vi "FullAlign.vi"(0 "Joystick 0":dbl, 1 "Button":bool=TRUE, 5 "Joystick 1":dbl, 7 "Distance":dbl=23.73829999999998, 9 "Angle":dbl=57.28800997198897) -> (4 "Right Motor":dbl, 6 "Left Motor":dbl=-0.0, 15 "In Range?":bool)   [LabVIEW 2016]
panel:
  in  "Range":dbl=25.0 step=5.0 format="%#_13g"
  out "Sees Target?":bool=TRUE
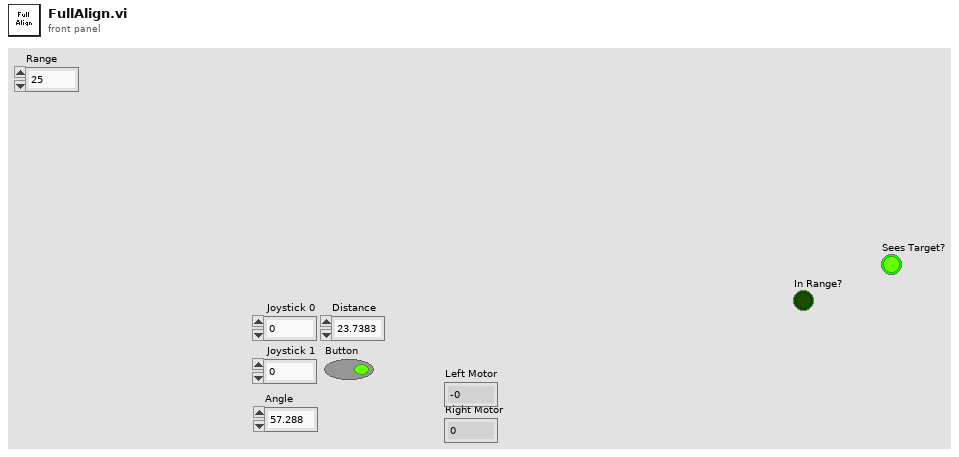
[diagram p1: front panel]
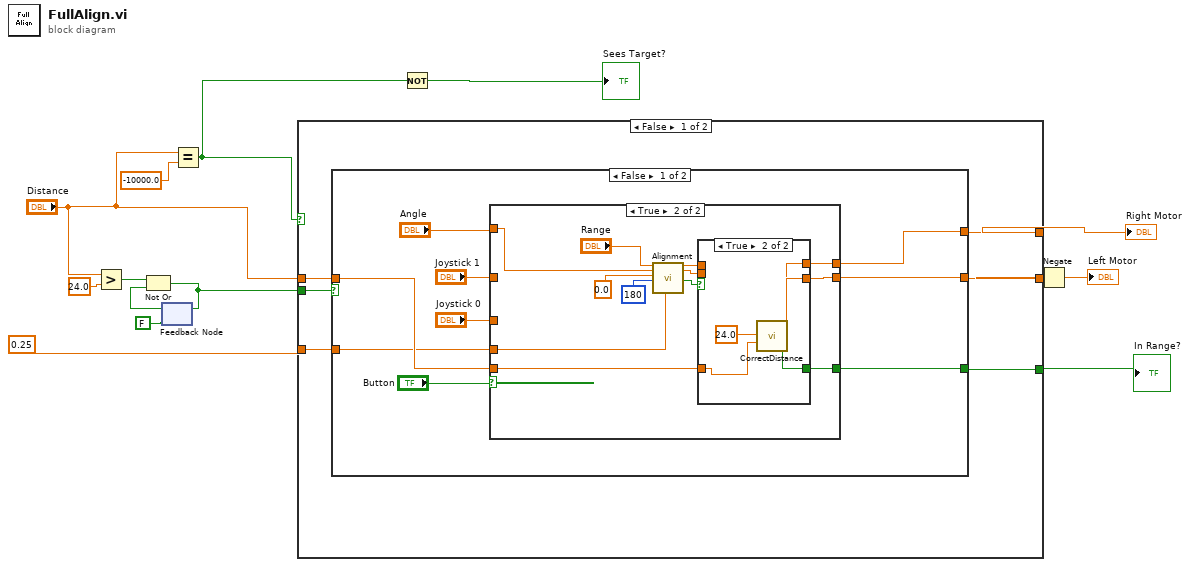
[diagram p0: block diagram]
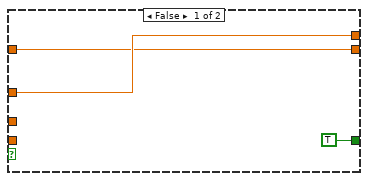
[diagram p2: hidden frame]
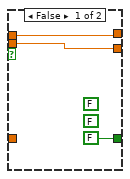
[diagram p3: hidden frame]
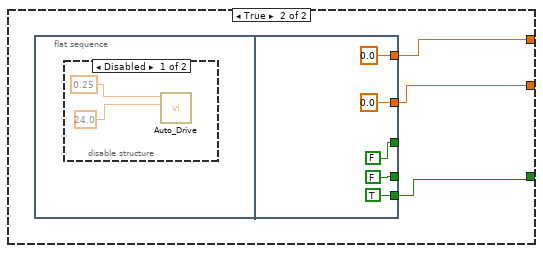
[diagram p4: hidden frame]
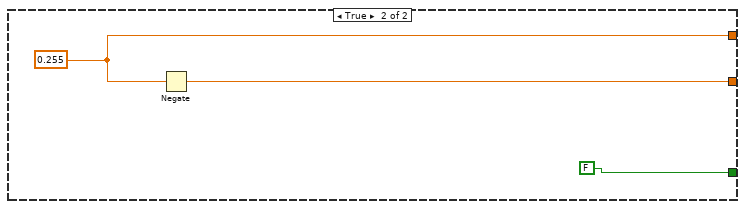
[diagram p6: hidden frame]
diagram:
  n1 = Greater?(x="Distance", y=24.0) -> (0:w11:bool)
  n2 = feedback #1(FALSE) -> (w12:bool)
  n3 = Not Or(1:w12, 2:w11) -> (0:w10:bool)
  n4 = feedback-in #1(w10) -> ()
  n5 = Equal?(x="Distance", y=-10000.0) -> (x = y?=w7:bool)
  n6 = case shown="False" w7 {
    tunnel: w10 -> [w20 _]
    tunnel: [w19 w63] -> w3
    tunnel: [w18 w64] -> w4
    tunnel: [w17 FALSE] -> w9
    tunnel: "Distance" -> [w16 _]
    tunnel: 0.25 -> [w15 _]
    frame False {
      n7 = case shown="False" w20 {
        tunnel: w16 -> [w25 _]
        tunnel: [w24 w54] -> w19
        tunnel: [w23 w53] -> w18
        tunnel: [w22 w55] -> w17
        tunnel: w15 -> [w21 _]
        frame False {
          n8 = case shown="True" "Button" {
            tunnel: "Joystick 1" -> [w31 _]
            tunnel: "Joystick 0" -> [w32 _]
            tunnel: [w31 w44] -> w23
            tunnel: [w32 w43] -> w24
            tunnel: "Angle" -> [_ w37]
            tunnel: [TRUE w42] -> w22
            tunnel: w25 -> [_ w41]
            tunnel: w21 -> [_ w36]
            frame False {
            }
            frame True {
              n9 = call "Alignment.vi"("Range"="Range", "Camera Feedback"=w37, "Target"=0.0, "POV"=180, "Turn_Gain"=w36) -> ("Right Motor"=w35:dbl, "Left Motor"=w34:dbl, "LeftAndRight?"=w33:bool)  [unwired: 12 in]
              n10 = case shown="True" w33 {
                tunnel: [w45 w51] -> w44
                tunnel: [w46 w50] -> w43
                tunnel: [FALSE w48] -> w42
                tunnel: w41 -> [_ w49]
                tunnel: w35 -> [w46 _]
                tunnel: w34 -> [w45 _]
                frame False {
                  (unwired) FALSE
                  (unwired) FALSE
                }
                frame True {
                  n11 = call "CorrectDistance.vi"("CenterPoint"=24.0, "Distance"=w49) -> ("In Range?"=w48:bool, "Right Motor"=w50:dbl, "Left Motor"=w51:dbl)  [unwired: 23 in]
                }
              }
            }
          }
        }
        frame True {
          n12 = flat-sequence {
            tunnel: [FALSE] -> _
            tunnel: [FALSE] -> _
            tunnel: [TRUE] -> w55
            tunnel: [0.0] -> w54
            tunnel: [0.0] -> w53
            frame #0 {
              n13 = disable-structure shown="Disabled" {
                frame Disabled {
                  n14 = call "Auto_Drive.vi"("distance"=24.0, "Drive Effort"=0.25) -> ()  [unwired: 10 in]
                }
                frame Enabled {
                }
              }
            }
            frame #1 {
            }
          }
        }
      }
    }
    frame True {
      w63 = 0.255
      n15 = Negate(x=w63) -> (-x=w64:dbl)
    }
  }
  "Right Motor" <- w3
  "In Range?" <- w9
  n16 = Not(x=w7) -> (.not. x?=→"Sees Target?":bool)
  n17 = Negate(x=w4) -> (-x=→"Left Motor":dbl)
